vi "Configure Trigger.vi"(6 "Operation Mode (0: Constant Current)":i32(ring) items=["Constant Current", "Constant Voltage"], 7 "Trigger Source (0: Immediately)":i32(ring) items=["Immediate", "Bus"], 8 "error in (no error)":errorcluster, 9 "Triggered Output Current (0)":dbl, 10 "Triggered Output Voltage (0)":dbl, 11 "VISA resource name":refnum<visa-resource-name>) -> (0 "error out":errorcluster, 3 "VISA resource name out":refnum<visa-resource-name>)   [LabVIEW 2023]
doc: "Configures the triggered output voltage, triggered output current, trigger source, and operation mode."
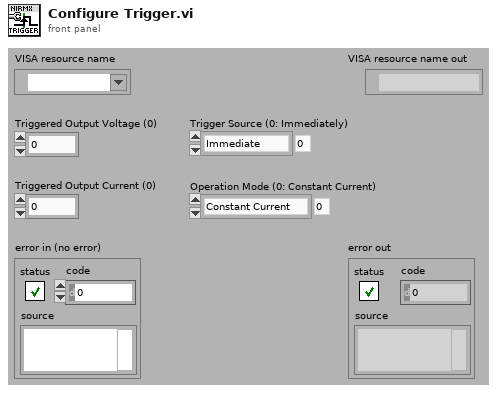
[diagram p1: front panel]
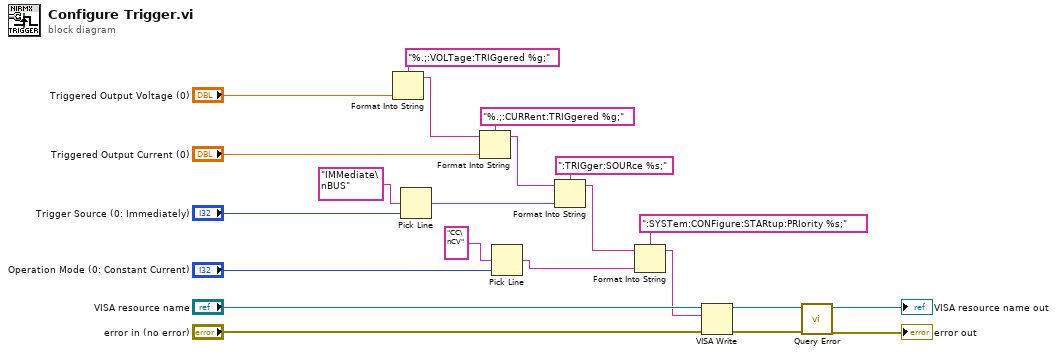
[diagram p0: block diagram]
diagram:
  n1 = Format Into String(format string="%.;:VOLTage:TRIGgered %g;", "Triggered Output Voltage (0)") -> (resulting string=w20:string)  [unwired: 2 in, 1 out]
  n2 = Pick Line(multi-line string="IMMediate\nBUS", line index="Trigger Source (0: Immediately)") -> (output string=w8:string)  [unwired: 1 in]
  n3 = Format Into String(format string="%.;:CURRent:TRIGgered %g;", initial string=w20, "Triggered Output Current (0)") -> (resulting string=w17:string)  [unwired: 1 in, 1 out]
  n4 = Pick Line(multi-line string="CC\nCV", line index="Operation Mode (0: Constant Current)") -> (output string=w5:string)  [unwired: 1 in]
  n5 = Format Into String(format string=":TRIGger:SOURce %s;", initial string=w17, w8) -> (resulting string=w2:string)  [unwired: 1 in, 1 out]
  n6 = Format Into String(format string=":SYSTem:CONFigure:STARtup:PRIority %s;", initial string=w2, w5) -> (resulting string=w3:string)  [unwired: 1 in, 1 out]
  n7 = VISA Write(VISA resource name="VISA resource name", write buffer=w3, error in (no error)="error in (no error)") -> (VISA resource name out=w13:refnum<visa-resource-name>, error out=w12:errorcluster)  [unwired: 1 out]
  n8 = call "Query Error.vi"("error in (no error)"=w12, "VISA resource name"=w13) -> ("error out"=→"error out":errorcluster, "VISA resource name out"=→"VISA resource name out":refnum<visa-resource-name>)  [unwired: 6 in, 2 out]
